vi "Picture Setup.vi"(8 "Error In":errorcluster, 10 "picture":picture, 11 "reference":refnum<vi>) -> (0 "Error Out":errorcluster)   [LabVIEW 2016]
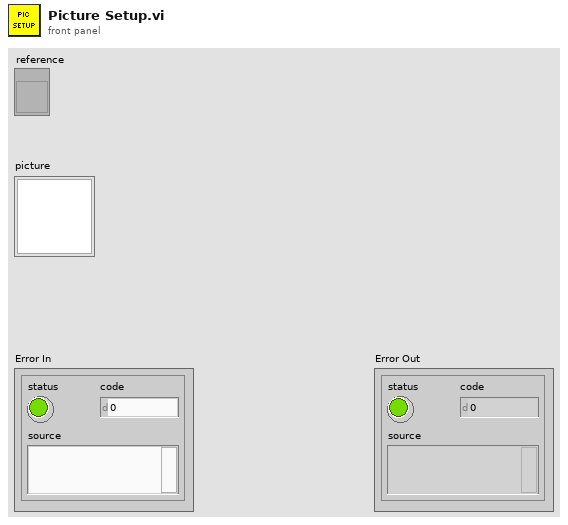
[diagram p1: front panel]
types:
  T1 = typedef "LVBoundsTypeDef.ctl" = cluster{"Width":u32, "Height":u32}
  T2 = typedef "imagedata.ctl" = cluster{"image type":i32, "image depth":i32, "image":u8[], "mask":u8[], "colors":u32[], "Rectangle":cluster{"left":i16, "top":i16, "right":i16, "bottom":i16}}
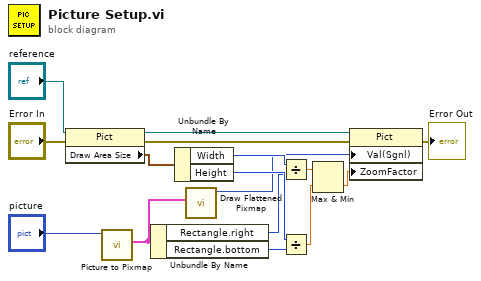
[diagram p0: block diagram]
diagram:
  n1 = property class="Pict"(reference="reference", error in="Error In") -> (reference out=w8:refnum<vi>, error out=w5:errorcluster, "Draw Area Size"=w9:T1)
  n2 = call <vilib>:"Picture to Pixmap.vi"("picture"="picture") -> ("image data"=w16:T2)  [unwired: 9 in, 1 out]
  n3 = Unbundle By Name(w16) -> ("Rectangle.right"=w11:i16, "Rectangle.bottom"=w13:i16)
  n4 = Unbundle By Name(w9) -> ("Width"=w10:u32, "Height"=w12:u32)
  n5 = call <vilib>:"Draw Flattened Pixmap.vi"("image data"=w16) -> ("new picture"=w6:picture)  [unwired: 8 in]
  n6 = Divide(x=w10, y=w11) -> (x/y=w14:dbl)
  n7 = Divide(x=w12, y=w13) -> (x/y=w15:dbl)
  n8 = Max & Min(x=w14, y=w15) -> (min(x,y)=w7:dbl)  [unwired: 1 out]
  n9 = property class="Pict"(reference=w8, error in=w5, "Val(Sgnl)"=w6, "ZoomFactor"=w7) -> (error out=→"Error Out":errorcluster)  [unwired: 1 out]
